vi "aft_xmpl_Simulate an Unknown System (Point By Point).vi"(8 "error in (no error)":errorcluster) -> (0 "error out":errorcluster, 1 "unknown system coefficients":dbl[](array[numeric])=[9.745429581298439e-18, 0.020461734458116075, 0.031830988618379075, 0.025008786559919588, -4.508492604200419e-17, -0.03215415414846812, -0.053051647697298455, -0.04501581580785527, 8.042442250270995e-17, 0.07502635967975894, 0.15915494309189543, 0.2250790790392766, 0.25, 0.2250790790392766, 0.15915494309189543, 0.07502635967975894, 8.042442250270995e-17, -0.04501581580785527, -0.053051647697298455, -0.03215415414846812, -4.508492604200419e-17, 0.025008786559919588, 0.031830988618379075, 0.020461734458116075, 9.745429581298439e-18], 2 "response signal":dbl, 3 "stimulus signal":dbl format="%0.2f")   [LabVIEW 2019]
doc: "Simulates the stimulus and response signals of an unknown system in point-by-point mode. This VI uses a lowpass FIR filter to simulate the unknown system. The input or stimulus to the unknown system is Gaussian white noise. The output or response of the unknown system is the input signal passing through the FIR filter."
uses:
  <vilib>/ptbypt/NI_PtbyPt.lvlib
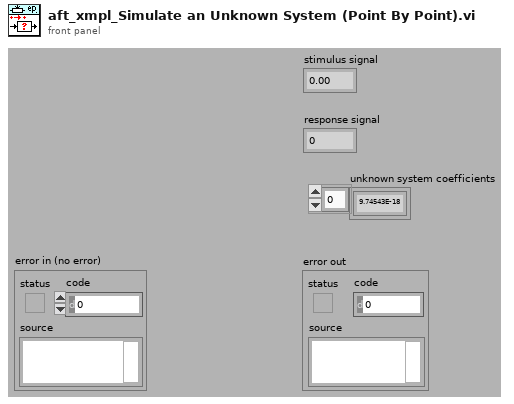
[diagram p1: front panel]
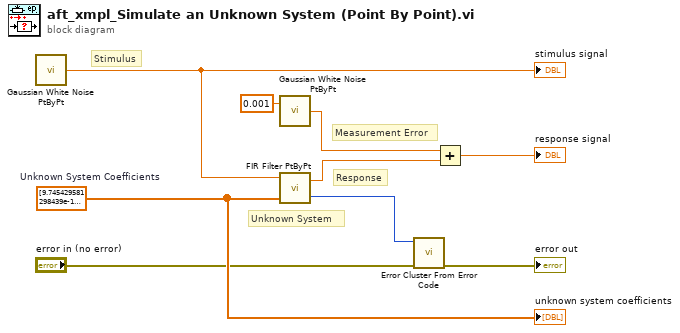
[diagram p0: block diagram]
diagram:
  w4 = dbl[] [9.745429581298439e-18, 0.020461734458116075, 0.031830988618379075, 0.025008786559919588, -4.508492604200419e-17, -0.03215415414846812, -0.053051647697298455, -0.04501581580785527, 8.042442250270995e-17, 0.07502635967975894, 0.15915494309189543, 0.2250790790392766, 0.25, 0.2250790790392766, 0.15915494309189543, 0.07502635967975894, 8.042442250270995e-17, -0.04501581580785527, -0.053051647697298455, -0.03215415414846812, -4.508492604200419e-17, 0.025008786559919588, 0.031830988618379075, 0.020461734458116075, 9.745429581298439e-18]  # Unknown System Coefficients
  # "Measurement Error"
  # "Stimulus"
  # "Response"
  # "Unknown System"
  n1 = call <vilib>:"Gaussian White Noise PtByPt.vi"() -> ("Gaussian white noise"=w6:dbl)  [unwired: 3 in]
  "stimulus signal" <- w6
  n2 = call <vilib>:"Gaussian White Noise PtByPt.vi"("standard deviation"=0.001) -> ("Gaussian white noise"=w8:dbl)  [unwired: 2 in]
  n3 = call <vilib>:"FIR Filter PtByPt.vi"("Forward Coefficients"=w4, "x"=w6) -> ("error"=w5:i32, "Filtered x"=w9:dbl)  [unwired: 1 in, 1 out]
  n4 = call <vilib>:"Error Cluster From Error Code.vi"("error in (no error)"="error in (no error)", "error code (0)"=w5) -> ("error out"=→"error out":errorcluster)  [unwired: 1 in, 6 out]
  n5 = Add(x=w8, y=w9) -> (x+y=→"response signal":dbl)
  "unknown system coefficients" <- w4
